vi "Write Representation.vi"(8 "error in (no error)":errorcluster, 10 "Rep":T1, 11 "Numeric.lvclass in":refnum<class "Numeric.lvclass">) -> (0 "error out":errorcluster, 3 "Numeric.lvclass out":refnum<class "Numeric.lvclass">)   [LabVIEW 2015, in "Numeric.lvclass"]
uses:
  Numeric.lvclass
  <vilib>/numeric/LVNumericRepresentation.ctl
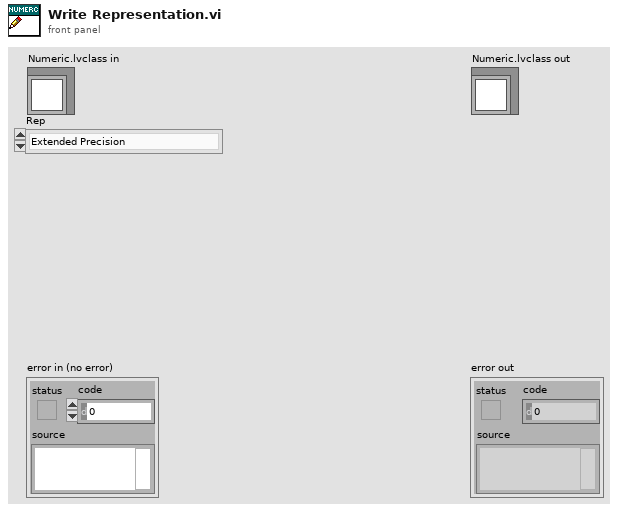
[diagram p1: front panel]
types:
  T1 = typedef "LVNumericRepresentation.ctl" = enum32{"Extended Precision", "Double Precision", "Single Precision", "Long", "Word", "Byte", "Unsigned Long", "Unsigned Word", "Unsigned Byte", "Complex Extended", "Complex Double", "Complex Single", "Quad", "Unsigned Quad", "Fixed-Point"}
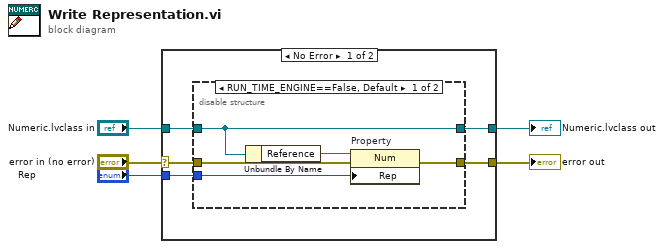
[diagram p0: block diagram]
diagram:
  n1 = case shown="No Error" "error in (no error)" {
    selector: "error in (no error)" -> [w6 w19]
    tunnel: [w10 w19] -> w4
    tunnel: [w7 w18] -> w2
    tunnel: "Numeric.lvclass in" -> [w8 w18]
    tunnel: "Rep" -> [w9 _]
    frame No Error {
      n2 = disable-structure shown="RUN_TIME_ENGINE==False, Default" {
        disable-tunnel: [w15 w16] -> w10
        disable-tunnel: w9 -> [w14 _]
        disable-tunnel: w8 -> [w12 w17]
        disable-tunnel: [w12 w17] -> w7
        disable-tunnel: w6 -> [w11 w16]
        frame condition #0 (active) {
          n3 = Unbundle By Name(w12) -> ("Reference"=w13:refnum<vi>)
          n4 = property on="Property" class="Num"(reference=w13, error in=w11, "Rep"=w14) -> (error out=w15:errorcluster)  [unwired: 1 out]
        }
        frame condition #1 {
        }
      }
    }
    frame Error {
    }
  }
  "error out" <- w4
  "Numeric.lvclass out" <- w2
